vi "Measure.vi"(8 "error in (no error)":errorcluster, 9 "measurement configuration":variant, 10 "measure call context in":refnum<class "Measure Call Context.lvclass">, 11 "measurement plugin in":refnum<class "FGEN Arb Sequence Mode.lvclass">) -> (0 "error out":errorcluster, 1 "measurement results":variant, 2 "measure call context out":refnum<class "Measure Call Context.lvclass">, 3 "measurement plugin out":refnum<class "FGEN Arb Sequence Mode.lvclass">)   [LabVIEW 2025, in "FGEN Arb Sequence Mode.lvclass"]
uses:
  FGEN Arb Sequence Mode.lvclass
  <vilib>/Plug-In SDKs/Measurements/Measure Call Context/Measure Call Context.lvclass
  Measurement Configuration.ctl
  FGEN Arb Sequence Mode.lvclass/FGEN Arb Sequence Mode.ctl
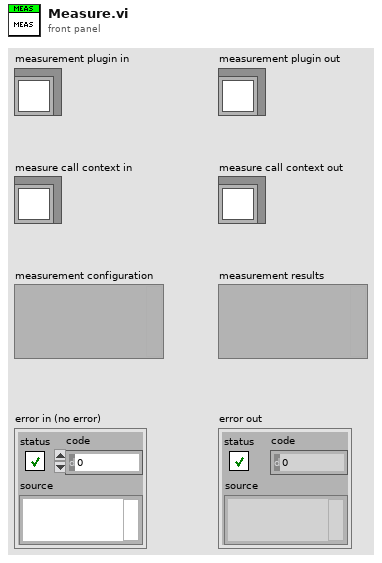
[diagram p1: front panel]
types:
  T1 = typedef "FGEN Arb Sequence Mode.lvclass/Measurement Configuration.ctl" = cluster{"TDMS File Path":string, "TDMS Channels":string[], "FGEN Resource Names":string[], "TDMS Groups":string[], "FGEN Waveform Names":string[], "Waveform Sequence":string[], "Loops Sequence":u32[], "Markers Sequence":i32[]}
  T2 = typedef "FGEN Arb Sequence Mode.lvclass/Measurement Results.ctl" = cluster{"Total Wfm Duration (s)":dbl, "FGEN Gain":dbl, "FGEN Sample Rate":dbl}
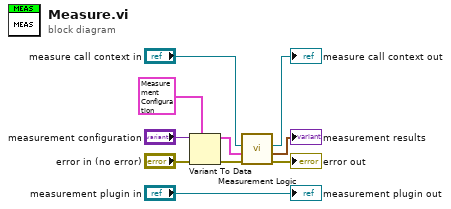
[diagram p0: block diagram]
diagram:
  n1 = Variant To Data(error in="error in (no error)", type=T1 {"TDMS File Path"="Lorem ipsum dolor sit", "TDMS Channels"=["", ""], "FGEN Resource Names"=["", ""], "TDMS Groups"=["", ""], "FGEN Waveform Names"=["", ""], "Waveform Sequence"=["", ""], "Loops Sequence"=[], "Markers Sequence"=[]} ("measurement configuration"), Variant="measurement configuration") -> (data=w1:T1, error out=w7:errorcluster)
  n2 = call "Measurement Logic.vi"("error in"=w7, "measurement configuration"=w1, "measure call context in"="measure call context in") -> ("error out"=→"error out":errorcluster, "measurement results"=→"measurement results":T2, "measure call context out"=→"measure call context out":refnum<class "Measure Call Context.lvclass">)  [unwired: 6 in]
  "measurement plugin out" <- "measurement plugin in"
